vi "测试专用.vi"(11 "JSON数据":string) -> (2 "值":string[](array[string]), 3 "键":string[](array[string]))   [LabVIEW 2014]
panel:
  out "错误输出":errorcluster caption="错误常量"
  in  "错误输入":errorcluster caption="错误常量"
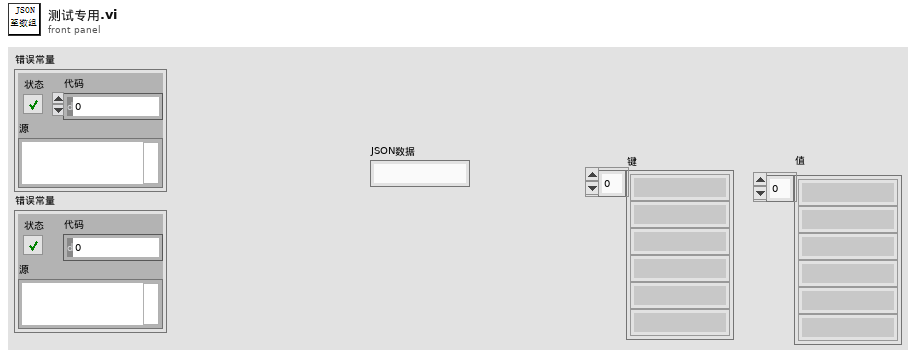
[diagram p1: front panel]
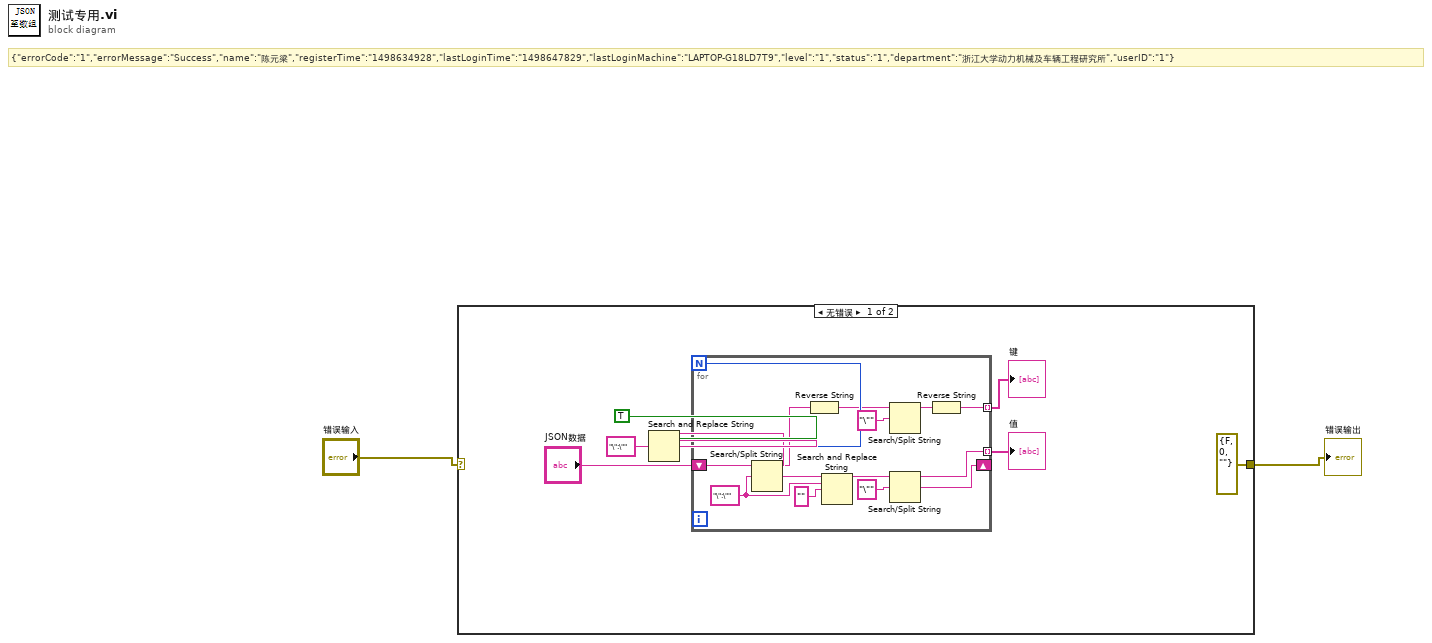
[diagram p0: block diagram]
diagram:
  # "{\"errorCode\":\"1\",\"errorMessage\":\"Success\",\"name\":\"陈元梁\",\"registerTime\":\"1498634928\",\"lastLoginTime\":\"1498647829\",\"lastLoginMachine\":\"LAPTOP-G18LD7T9\",\"level\":\"1\",\"status\":\"1\",\"department\":\"浙江大学动力机械及车辆工程研究所\",\"userID\":\"1\"}"
  n1 = case shown="无错误" "错误输入" {
    selector: "错误输入" -> [_ w23]
    tunnel: [errorcluster {"status"=FALSE, "code"=0, "source"=""} ("error IO") w23] -> w1
    frame No Error {
      n2 = Search and Replace String(replace all?=TRUE ("替换全部？(F)"), input string="JSON数据", search string="\":\"" ("搜索字符串")) -> (number of replacements=w6:i32)  [unwired: 5 in, 3 out]
      n3 = for {
        N: w6 -> [_]
        shift-right: [w12] -> _
        shift-left: "JSON数据" -> [w22]
        tunnel: [w11] -> w5 mode=indexing
        tunnel: [w10] -> w4 mode=indexing
        w20 = "\":\"" ("搜索字符串")
        n4 = Search/Split String(string=w22, search string/char (-)=w20) -> (substring before match=w18:string, match + rest of string=w21:string)  [unwired: 1 in, 1 out]
        n5 = Reverse String(1:w18) -> (0:w17:string)
        n6 = Search and Replace String(input string=w21, search string=w20, replace string="" ("替换字符串(\"\")")) -> (result string=w13:string)  [unwired: 5 in, 3 out]
        n7 = Search/Split String(string=w17, search string/char (-)="\"" ("搜索字符串/字符(-)")) -> (substring before match=w15:string)  [unwired: 1 in, 2 out]
        n8 = Search/Split String(string=w13, search string/char (-)="\"" ("搜索字符串/字符(-)")) -> (substring before match=w10:string, match + rest of string=w12:string)  [unwired: 1 in, 1 out]
        n9 = Reverse String(1:w15) -> (0:w11:string)
      }
      "键" <- w5
      "值" <- w4
    }
    frame Error {
    }
  }
  "错误输出" <- w1
